vi "ARD-LTC2499_Example.vi"   [LabVIEW 2014]
uses:
  QwaveSys_ESP8266/QwaveSys_ESP8266.lvlib
  QwaveSys_Interface/QwaveSys_Interface.lvlib
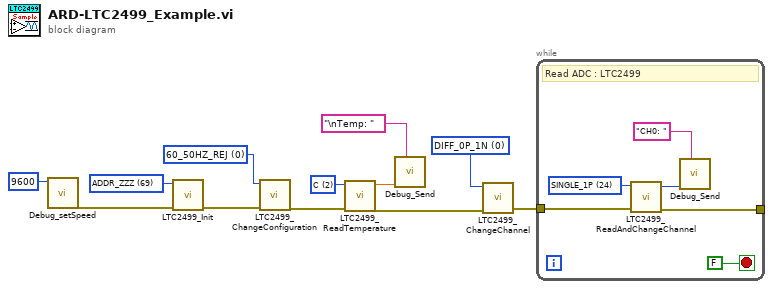
[diagram p0: block diagram]
diagram:
  w9 = u16 2 items=["K", "F", "C"] ("Temp Type")
  w3 = u16 0 items=["TEMPERATURE"=64, "SINGLE_0P"=16, "SINGLE_1P"=24, "SINGLE_2P"=17, "SINGLE_3P"=25, "SINGLE_4P"=18, "SINGLE_5P"=26, "SINGLE_6P"=19, "SINGLE_7P"=27, "SINGLE_8P"=20, "SINGLE_9P"=28, "SINGLE_10P"=21, "SINGLE_11P"=29, "SINGLE_12P"=22, "SINGLE_13P"=30, "SINGLE_14P"=23, "SINGLE_15P"=31, "DIFF_0P_1N"=0, "DIFF_2P_3N"=1, "DIFF_4P_5N"=2, "DIFF_6P_7N"=3, "DIFF_8P_9N"=4, "DIFF_10P_11N"=5, "DIFF_12P_13N"=6, "DIFF_14P_15N"=7, "DIFF_1P_0N"=8, "DIFF_3P_2N"=9, "DIFF_5P_4N"=10, "DIFF_7P_6N"=11, "DIFF_9P_8N"=12, "DIFF_11P_10N"=13, "DIFF_13P_12N"=14, "DIFF_15P_14N"=15] ("Channel")
  w10 = u16 0 items=["60_50HZ_REJ"=0, "60HZ_REJ"=32, "50HZ_REJ"=16, "SPEED_2X"=8] ("Config")
  w12 = u8 69 items=["ADDR_000"=20, "ADDR_00Z"=21, "ADDR_001"=22, "ADDR_0Z0"=23, "ADDR_0ZZ"=36, "ADDR_0Z1"=37, "ADDR_010"=38, "ADDR_01Z"=39, "ADDR_011"=40, "ADDR_Z00"=53, "ADDR_Z01"=55, "ADDR_Z0Z"=54, "ADDR_ZZ0"=68, "ADDR_ZZZ"=69, "ADDR_ZZ1"=70, "ADDR_Z10"=71, "ADDR_Z1Z"=84, "ADDR_Z11"=85, "ADDR_100"=86, "ADDR_10Z"=87, "ADDR_101"=100, "ADDR_1Z0"=101, "ADDR_1ZZ"=102, "ADDR_1Z1"=103, "ADDR_110"=116, "ADDR_111"=117, "ADDR_11Z"=118] ("Address")
  n1 = call "Debug_setSpeed.vi"("Speed"=u32 9600) -> ("error out"=w5:errorcluster)  [unwired: 10 in]
  n2 = call "LTC2499_Init.vi"("error in (no error)"=w5, "Address"=w12) -> ("error out"=w11:errorcluster)  [unwired: 9 in]
  n3 = call "LTC2499_ChangeConfiguration.vi"("error in (no error)"=w11, "Config"=w10) -> ("error out"=w4:errorcluster)  [unwired: 9 in]
  n4 = call "LTC2499_ReadTemperature.vi"("error in (no error)"=w4, "Temp Type"=w9) -> ("error out"=w1:errorcluster, "Data"=w8:dbl)  [unwired: 8 in]
  n5 = call "Debug_Send.vi"("Name"="\nTemp: ", "DATA"=w8) -> ()  [unwired: 10 in]
  n6 = call "LTC2499_ChangeChannel.vi"("error in (no error)"=w1, "Channel"=w3) -> ("error out"=w2:errorcluster)  [unwired: 9 in]
  n7 = while {
    tunnel: w2 -> [w16]
    tunnel: [w13] -> _
    stop <- FALSE stop-if-true
    w14 = u16 24 items=["TEMPERATURE"=64, "SINGLE_0P"=16, "SINGLE_1P"=24, "SINGLE_2P"=17, "SINGLE_3P"=25, "SINGLE_4P"=18, "SINGLE_5P"=26, "SINGLE_6P"=19, "SINGLE_7P"=27, "SINGLE_8P"=20, "SINGLE_9P"=28, "SINGLE_10P"=21, "SINGLE_11P"=29, "SINGLE_12P"=22, "SINGLE_13P"=30, "SINGLE_14P"=23, "SINGLE_15P"=31, "DIFF_0P_1N"=0, "DIFF_2P_3N"=1, "DIFF_4P_5N"=2, "DIFF_6P_7N"=3, "DIFF_8P_9N"=4, "DIFF_10P_11N"=5, "DIFF_12P_13N"=6, "DIFF_14P_15N"=7, "DIFF_1P_0N"=8, "DIFF_3P_2N"=9, "DIFF_5P_4N"=10, "DIFF_7P_6N"=11, "DIFF_9P_8N"=12, "DIFF_11P_10N"=13, "DIFF_13P_12N"=14, "DIFF_15P_14N"=15] ("Next Channel")
    # "Read ADC : LTC2499"
    n8 = call "LTC2499_ReadAndChangeChannel.vi"("error in (no error)"=w16, "Next Channel"=w14) -> ("error out"=w13:errorcluster, "Data"=w15:i32)  [unwired: 8 in]
    n9 = call "Debug_Send.vi"("Name"="CH0: ", "DATA"=w15) -> ()  [unwired: 10 in]
  }
